vi "AudioStreamer.Close.vi"() -> (0 "success":bool)   [LabVIEW 2020]
uses:
  <vilib>/Utility/sysdir.llb/System Directory Type.ctl
  <vilib>/Utility/config.llb/Write Key (I32).vi
  <vilib>/Utility/config.llb/NI_LVConfig.lvlib
panel:
  out "error out":errorcluster
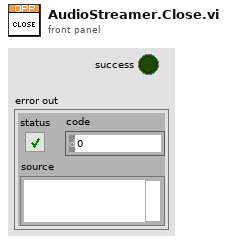
[diagram p1: front panel]
types:
  T1 = enum32{"Bad", "Idle", "Run top level", "Running"}
  T2 = typedef "System Directory Type.ctl" = i32
  T3 = typedef "LVRectTypeDef.ctl" = cluster{"Left":i16, "Top":i16, "Right":i16, "Bottom":i16}
  T4 = typedef "NI_LVConfig.lvlib/Config Data RefNum.ctl" = refnum<k1>
  T5 = enum32{"Invalid", "Standard", "Closed", "Hidden", "Minimized", "Maximized"}
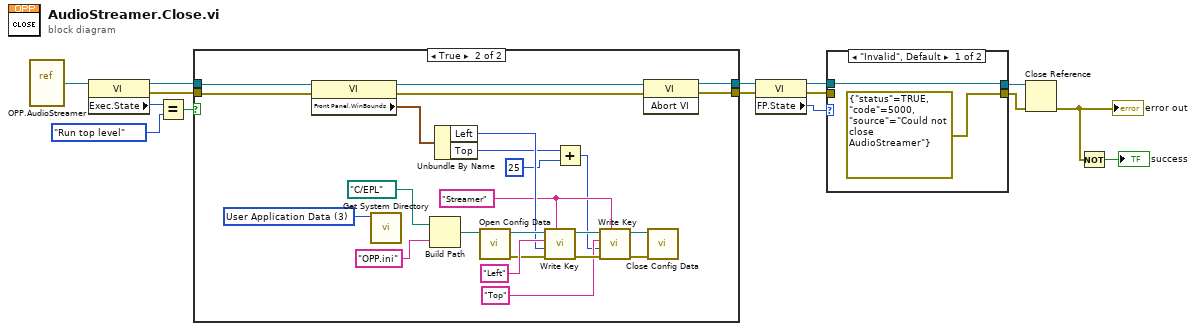
[diagram p0: block diagram]
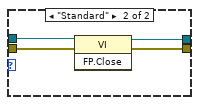
[diagram p2: hidden frame]
diagram:
  n1 = vi-ref "OPP.AudioStreamer.vi"() -> (w12:refnum<vi>)
  n2 = property class="VI"(reference=w12) -> (reference out=w15:refnum<vi>, error out=w14:errorcluster, "Exec.State"=w11:T1)  [unwired: 1 in]
  n3 = Equal?(x=w11, y=T1."Run top level" ("Execution:State")) -> (x = y?=w10:bool)
  n4 = case shown="True" w10 {
    tunnel: w15 -> [w17 w21]
    tunnel: w14 -> [w16 w20]
    tunnel: [w17 w41] -> w7
    tunnel: [w16 w40] -> w6
    frame False {
    }
    frame True {
      w29 = "Streamer" ("section")
      w38 = T2 3 items=["User Home"=0, "User Desktop"=1, "User Documents"=2, "User Application Data"=3, "User Preferences"=4, "User Temporary"=5, "Public Documents"=6, "Public Application Data"=7, "Public Preferences"=8, "Public Cache"=13, "System Core Libraries"=9, "System Installed Libraries"=10, "Application Files"=11, "Boot Volume Root"=12] ("system directory type")
      n5 = property class="VI"(reference=w21, error in=w20) -> (reference out=w19:refnum<vi>, error out=w18:errorcluster, "Front Panel.WinBounds"=w39:T3)
      n6 = call <vilib>:"Get System Directory.vi"("system directory type"=w38) -> ()  [unwired: 10 in, 1 out]
      n7 = Build Path(base path=path "C:/EPL", name or relative path="OPP.ini") -> (appended path=w36:path)
      n8 = Unbundle By Name(w39) -> ("Left"=w33:i16, "Top"=w28:i16)
      n9 = call <vilib>:"Open Config Data.vi"("configuration file path"=w36) -> ("error out"=w31:errorcluster, "refnum"=w35:T4)  [unwired: 8 in, 1 out]
      n10 = call-poly <vilib>:"Write Key.vi"("section"=w29, "error in (no error)"=w31, "value"=w33, "key"="Left", "refnum"=w35) -> ("error out"=w30:errorcluster, "refnum out"=w32:T4)  [unwired: 4 in, 1 out]
      n11 = Add(x=w28, y=i16 25) -> (x+y=w24:i16)
      n12 = call-poly <vilib>:"Write Key.vi"("section"=w29, "error in (no error)"=w30, "value"=w24, "key"="Top", "refnum"=w32) -> ("error out"=w26:errorcluster, "refnum out"=w25:T4)  [unwired: 4 in, 1 out]
      n13 = invoke class="VI" method="Abort VI"(reference=w19, error in=w18) -> (reference out=w41:refnum<vi>, error out=w40:errorcluster)  [unwired: 1 in, 1 out]
      n14 = call <vilib>:"Close Config Data.vi"("error in (no error)"=w26, "refnum"=w25) -> ()  [unwired: 8 in, 2 out]
    }
  }
  n15 = property class="VI"(reference=w7, error in=w6) -> (reference out=w5:refnum<vi>, error out=w1:errorcluster, "FP.State"=w4:T5)
  n16 = case shown="\"Invalid\", Default" w4 {
    tunnel: [w42 w47] -> w3
    tunnel: [errorcluster {"status"=TRUE, "code"=5000, "source"="Could not close AudioStreamer"} ("error out") w46] -> w2
    tunnel: w5 -> [w42 w45]
    tunnel: w1 -> [_ w44]
    frame "Invalid", Default {
    }
    frame "Standard" {
      n17 = invoke class="VI" method="FP.Close"(reference=w45, error in=w44) -> (reference out=w47:refnum<vi>, error out=w46:errorcluster)  [unwired: 1 in, 1 out]
    }
  }
  n18 = Close Reference(reference=w3, error in (no error)=w2) -> (error out=w8:errorcluster)
  "error out" <- w8
  n19 = Not(x=w8) -> (.not. x?=→"success":bool)
